vi "Connect.vi"(6 "Access (R/W allowed)":T1, 8 "error in (no error)":errorcluster, 11 "PVConnection in":refnum<class "SVConnection.lvclass">) -> (0 "error out":errorcluster, 3 "PVConnection out":refnum<class "SVConnection.lvclass">)   [LabVIEW 2013, in "CS++ProcessVariables.lvlib" / "SVConnection.lvclass"]
doc: "Opene reference to a shared variable if not already connected."
uses:
  SVConnection.lvclass
  SVConnection.lvclass/SVConnection.ctl
  PVConnection/PVConnection.lvclass/PVConnection.ctl
  ProcessVariable/PV.lvclass/PV.ctl
  ProcessVariable/PV.lvclass
  PVConnection/PVConnection.lvclass
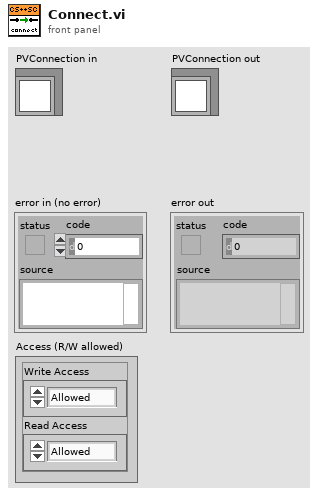
[diagram p1: front panel]
types:
  T1 = cluster{"Write Access":enum8{"Allowed", "Required", "None"}, "Read Access":enum8{"Allowed", "Required", "None"}}
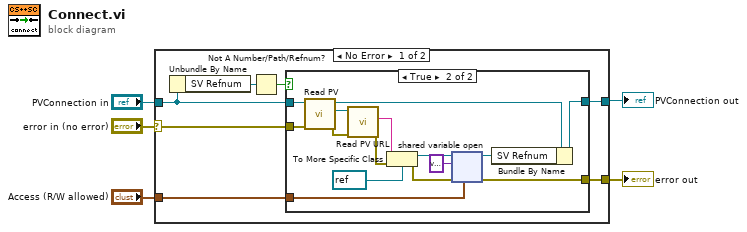
[diagram p0: block diagram]
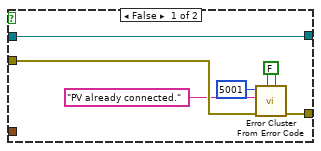
[diagram p2: hidden frame]
diagram:
  n1 = case shown="No Error" "error in (no error)" {
    selector: "error in (no error)" -> [w12 w35]
    tunnel: [w11 w35] -> w4
    tunnel: [w10 w34] -> w2
    tunnel: "PVConnection in" -> [w6 w34]
    tunnel: "Access (R/W allowed)" -> [w7 _]
    frame No Error {
      n2 = Unbundle By Name(w6) -> ("SV Refnum"=w9:refnum<k21>)
      n3 = Not A Number/Path/Refnum?(number/path/refnum=w9) -> (NaN/Path/Refnum?=w8:bool)
      n4 = case shown="True" w8 {
        tunnel: w12 -> [w17 w20]
        tunnel: [w16 w29] -> w11
        tunnel: [w18 w27] -> w10
        tunnel: w6 -> [w18 w24]
        tunnel: w7 -> [_ w26]
        frame False {
          w15 = FALSE ("show call chain? (False)")
          n5 = call <vilib>:"Error Cluster From Error Code.vi"("is warning? (False)"=w15, "show call chain? (False)"=w15, "error in (no error)"=w17, "error message (\"\")"="PV already connected." ("error message (\"\")"), "error code (0)"=5001) -> ("error out"=w16:errorcluster)  [unwired: 4 in]
        }
        frame True {
          n6 = call "Read PV.vi"("error in (no error)"=w20, "PVConnection in"=w24) -> ("error out"=w22:errorcluster, "PV"=w23:refnum<class "PV.lvclass">, "PVConnection out"=w19:refnum<class "SVConnection.lvclass">)  [unwired: 7 in]
          n7 = call "Read PV URL.vi"("error in (no error)"=w22, "PV in"=w23) -> ("error out"=w21:errorcluster, "PV URL"=w25:string)  [unwired: 7 in, 1 out]
          n8 = To More Specific Class(target class=refnum<k21> refnum ("shared variable refnum in"), reference=w25, error in=w21) -> (specific class reference=w32:refnum<k21>, error out=w31:errorcluster)
          n9 = shared-variable-open(w32, w31, variant ("variant"), w26) -> (w28:refnum<k21>, w29:errorcluster)
          n10 = Bundle By Name(cluster=w19, "SV Refnum"=w28) -> (w27:refnum<class "SVConnection.lvclass">)
        }
      }
    }
    frame Error {
    }
  }
  "error out" <- w4
  "PVConnection out" <- w2
